vi "Pre Launch Init.vi"(11 "Power Supply in":refnum<class "Power Supply.lvclass">) -> (0 "error out":errorcluster, 3 "Power Supply out":refnum<class "Power Supply.lvclass">)   [LabVIEW 2020, in "Power Supply.lvlib" / "Power Supply.lvclass"]
doc: "(<B>Filename</B>: Actor Framework.lvlib:Actor.lvclass:Pre Launch Init.vi)\n\nDefines behavior that occurs after the Launch Nested Actor method is invoked but before the actor's Actor Core method begins running.\n\nBy default, this method does nothing. A descendant class may override it to define behavior."
uses:
  Power Supply.lvclass
  Power Supply.lvclass/Power Supply.ctl
  <vilib>/ActorFramework/Actor/Actor.lvclass
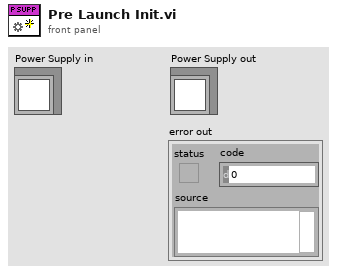
[diagram p1: front panel]
types:
  T1 = cluster{"Output Status":refnum<user-event>, "Stop":refnum<user-event>, "Status":refnum<user-event>}
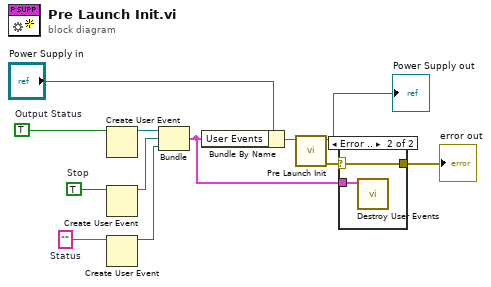
[diagram p0: block diagram]
diagram:
  w8 = ""  # Status
  w9 = TRUE  # Stop
  w10 = TRUE  # Output Status
  n1 = Create User Event(user event datatype=w10) -> (user event=w7:refnum<user-event>)  [unwired: 1 in, 1 out]
  n2 = Create User Event(user event datatype=w9) -> (user event=w6:refnum<user-event>)  [unwired: 1 in, 1 out]
  n3 = Create User Event(user event datatype=w8) -> (user event=w5:refnum<user-event>)  [unwired: 1 in, 1 out]
  n4 = Bundle("Output Status"=w7, "Stop"=w6, "Status"=w5) -> (w1:T1)  [unwired: 1 in]
  n5 = Bundle By Name(cluster="Power Supply in", "User Events"=w1) -> (w4:refnum<class "Power Supply.lvclass">)
  n6 = call-parent "Pre Launch Init.vi"("Actor in"=w4) -> ("error out"=w3:errorcluster, "Actor out"=→"Power Supply out":refnum<class "Power Supply.lvclass">)  [unwired: 9 in]
  n7 = case shown="Error .." w3 {
    selector: w3 -> [w13 w14]
    tunnel: [w13 w14] -> w2
    tunnel: w1 -> [_ w15]
    frame No Error {
    }
    frame Error {
      n8 = call "Destroy User Events.vi"("Cluster"=w15) -> ()  [unwired: 11 in]
    }
  }
  "error out" <- w2
